vi "Kinesis - BNT - Set Circle Home Position.vi"() -> ()   [LabVIEW 2012]
doc: "Shows how to set and get the NanoTrak circle home position."
uses:
  U:/Kinesis LabVIEW Website Examples/Thorlabs.MotionControl.Controls.dll
  Thorlabs.MotionControl.Controls.dll
  U:/Kinesis LabVIEW Website Examples/Thorlabs.MotionControl.Benchtop.NanoTrakCLI.dll
  Thorlabs.MotionControl.Benchtop.NanoTrakCLI.dll
  U:/Kinesis LabVIEW Website Examples/Thorlabs.MotionControl.GenericNanoTrakCLI.dll
  Thorlabs.MotionControl.GenericNanoTrakCLI.dll
panel:
  in  "?":bool
  in  "Set Position":cluster{"HPosition":dbl, "VPosition":dbl}
  out "New Position":cluster{"HPosition":dbl, "VPosition":dbl}
  in  "?":bool
  out "Initial Position":cluster{"HPosition":dbl, "VPosition":dbl}
  in  "SerialNumber":string
  in  "BenchtopNanoTrakControl":refnum<k24>(container)
  # "Notes:"
  # "- Ensure that the appropriate .DLLs are copied into your Project Folder. Check that the correct bit type are used depending on your version of LabVIEW\ni.e. 32-bit or 64-bit.\n\n\n\n\n\n\n\n\n\n\n\n\n\n\n- Open the example VI through the LabVIEW Project Explorer to correctly load the User Interface from Thorlabs.MotionControl.Controls.dll."
  # "Thorlabs Hardware: BNT001/IR\nhttps://www.thorlabs.com/newgrouppage9.cfm?objectgroup_id=1194&pn=BNT001/IR"
  # "Description: This VI will enable you to set the Scanning Circle Home Position, throught the GetCircleHomePosition() method. \nHorizontal and Vertical positions can be adjusted in the range of 0 to 10 in NanoTrak Units."
  # "Instructions: \n1) Connect your BNT001 device to your PC & power the device. For full device setup, the device product manual can be found on our website here.\n - https://www.thorlabs.com/thorproduct.cfm?partnumber=BNT001/IR\n2) Enter the device serial number below.\n3) Click 'Run' in the LabVIEW Toolbar.\n5) Enter values for Horizontal & Vertical Position (0-10 NT Units). \n5) To end the Program, click 'END'."
  # "Example Image of .NET Controller - VI opened via Project Explorer/ not opened via Project Explorer"
  # "VI Not Opened via Project Explorer"
  # "VI Opened via Project Explorer"
  # "- To explore the range of methods available, please visit the .NET API, included with your Kinesis software.\n\n- For tips on building your own VIs with Thorlabs Motion Control Hardware, please see our LabVIEW Guide here.\nhttps://www.thorlabs.com/newgrouppage9.cfm?objectgroup_id=10285"
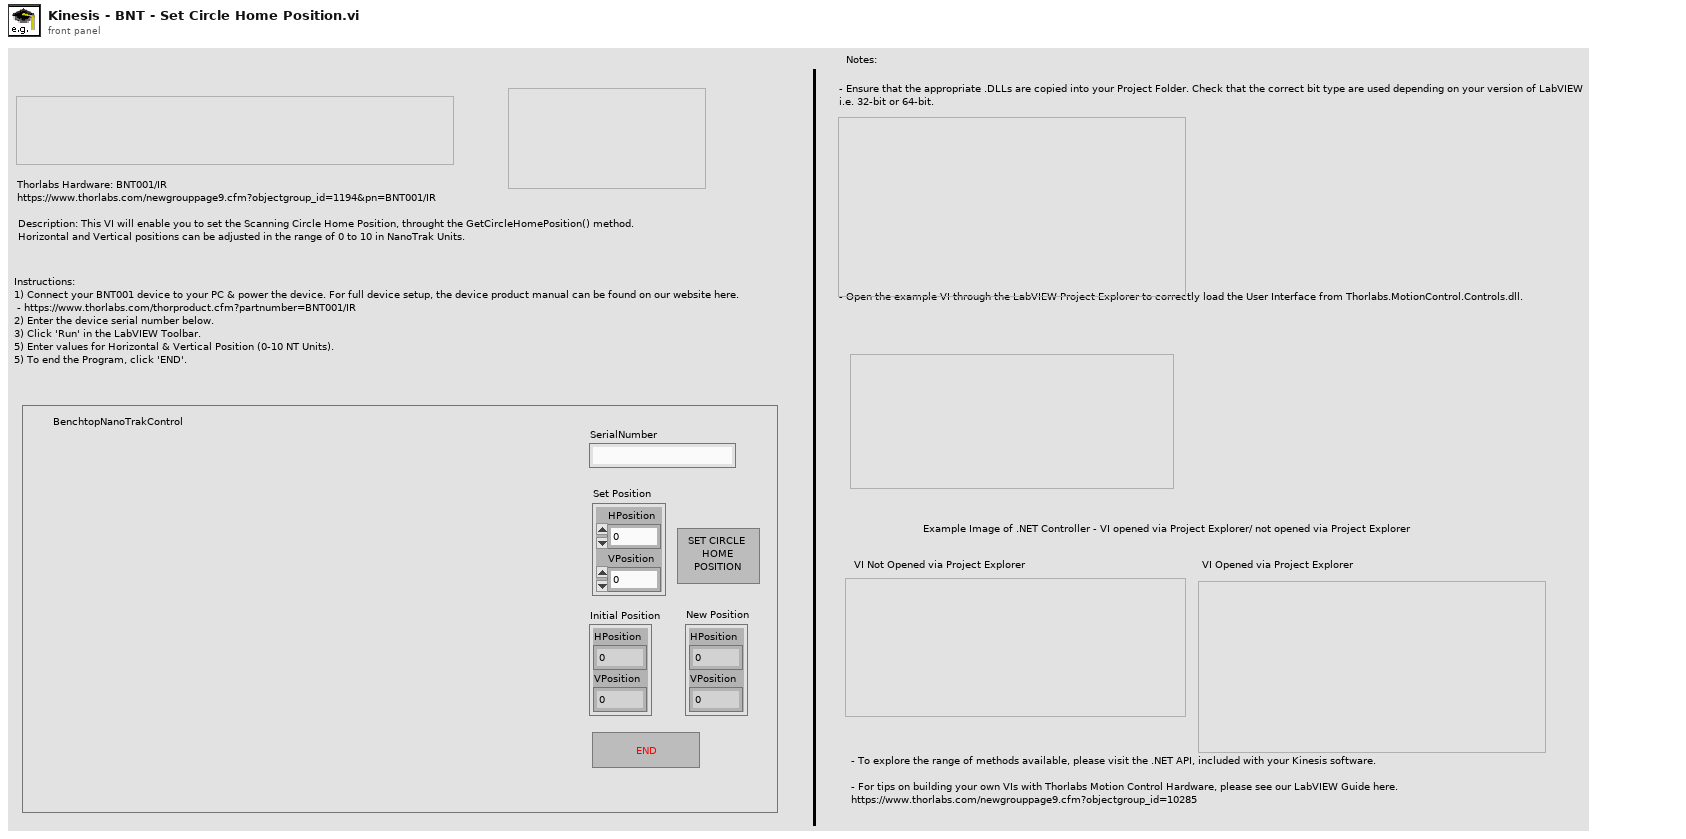
[diagram p1: front panel]
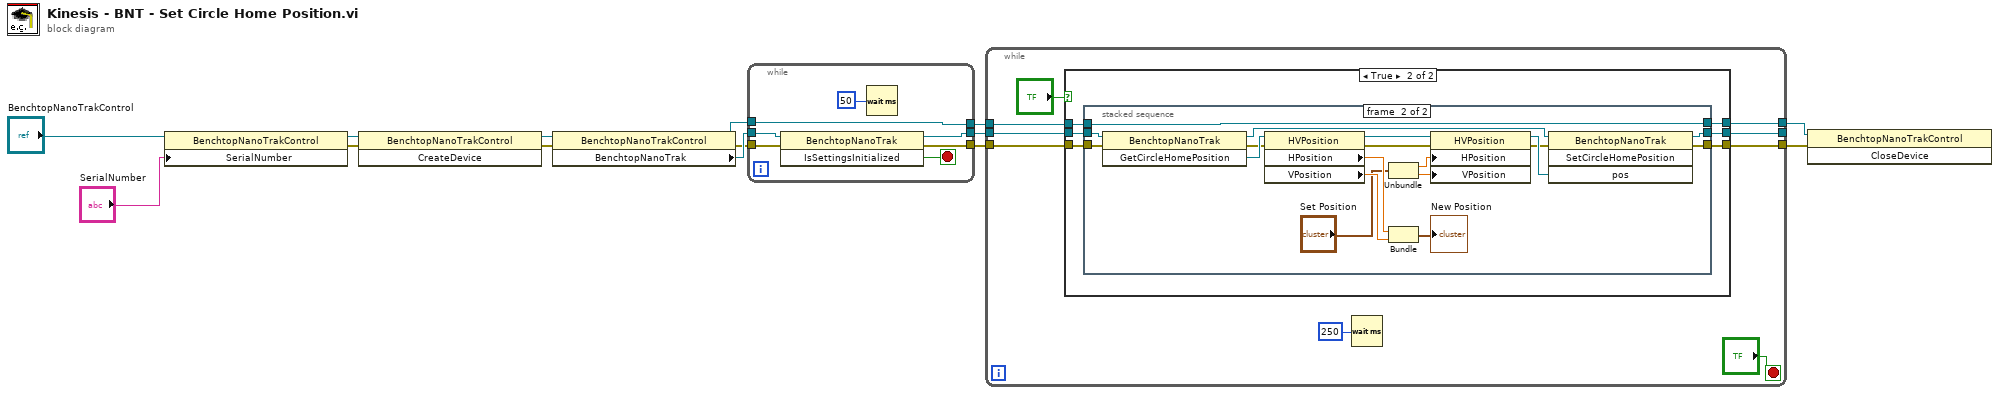
[diagram p0: block diagram]
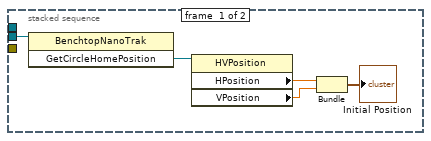
[diagram p3: hidden frame]
diagram:
  n1 = property class="BenchtopNanoTrakControl"(reference="BenchtopNanoTrakControl", "SerialNumber"="SerialNumber") -> (reference out=w12:refnum<k24>, error out=w7:errorcluster)  [unwired: 1 in]
  n2 = invoke class="BenchtopNanoTrakControl" method="CreateDevice"(reference=w12, error in=w7) -> (reference out=w11:refnum<k24>, error out=w8:errorcluster)  [unwired: 1 in, 1 out]
  n3 = property class="BenchtopNanoTrakControl"(reference=w11, error in=w8) -> (reference out=w1:refnum<k24>, error out=w9:errorcluster, "BenchtopNanoTrak"=w10:refnum<k24>)
  n4 = while {
    tunnel: w10 -> [w19]
    tunnel: [w18] -> w5
    tunnel: w9 -> [w17]
    tunnel: [w16] -> w6
    tunnel: [w15] -> w2
    tunnel: w1 -> [w15]
    stop <- w21 stop-if-true
    n5 = invoke class="BenchtopNanoTrak" method="IsSettingsInitialized"(reference=w19, error in=w17) -> (reference out=w18:refnum<k24>, error out=w16:errorcluster, "IsSettingsInitialized"=w21:bool)  [unwired: 1 in]
    n6 = Wait (ms)(milliseconds to wait=u32 50) -> ()  [unwired: 1 out]
  }
  n7 = while {
    tunnel: [w25] -> _
    tunnel: w6 -> [w28]
    tunnel: [w27] -> w4
    tunnel: w5 -> [w26]
    tunnel: [w24] -> w3
    tunnel: w2 -> [w23]
    stop <- "?" stop-if-true
    n8 = case shown="True" "?" {
      tunnel: w26 -> [w32 w39]
      tunnel: [w32 w38] -> w25
      tunnel: w28 -> [w33 w37]
      tunnel: [w33 w36] -> w27
      tunnel: [w31 w35] -> w24
      tunnel: w23 -> [w31 w34]
      frame False {
      }
      frame True {
        n9 = stacked-sequence {
          tunnel: w39 -> [w44 w58]
          tunnel: [_ w51] -> w38
          tunnel: w37 -> [_ w50]
          tunnel: [_ w46] -> w36
          tunnel: [_ w45] -> w35
          tunnel: w34 -> [_ w45]
          frame #0 {
            n10 = invoke class="BenchtopNanoTrak" method="GetCircleHomePosition"(reference=w44) -> ("GetCircleHomePosition"=w43:refnum<k24>)  [unwired: 2 in, 2 out]
            n11 = property class="HVPosition"(reference=w43) -> ("HPosition"=w42:dbl, "VPosition"=w41:dbl)  [unwired: 1 in, 2 out]
            n12 = Bundle("HPosition"=w42, "VPosition"=w41) -> (→"Initial Position":cluster{"HPosition":dbl, "VPosition":dbl})  [unwired: 1 in]
          }
          frame #1 {
            n13 = invoke class="BenchtopNanoTrak" method="GetCircleHomePosition"(reference=w58, error in=w50) -> (reference out=w52:refnum<k24>, error out=w49:errorcluster, "GetCircleHomePosition"=w62:refnum<k24>)  [unwired: 1 in]
            n14 = property class="HVPosition"(reference=w62, error in=w49) -> (reference out=w53:refnum<k24>, error out=w48:errorcluster, "HPosition"=w61:dbl, "VPosition"=w60:dbl)
            n15 = Unbundle("Set Position") -> ("HPosition"=w56:dbl, "VPosition"=w55:dbl)
            n16 = Bundle("HPosition"=w61, "VPosition"=w60) -> (→"New Position":cluster{"HPosition":dbl, "VPosition":dbl})  [unwired: 1 in]
            n17 = property class="HVPosition"(reference=w53, error in=w48, "HPosition"=w56, "VPosition"=w55) -> (reference out=w54:refnum<k24>, error out=w47:errorcluster)
            n18 = invoke class="BenchtopNanoTrak" method="SetCircleHomePosition"(reference=w52, error in=w47, "pos"=w54) -> (reference out=w51:refnum<k24>, error out=w46:errorcluster)  [unwired: 1 in, 2 out]
          }
        }
      }
    }
    n19 = Wait (ms)(milliseconds to wait=u32 250) -> ()  [unwired: 1 out]
  }
  n20 = invoke class="BenchtopNanoTrakControl" method="CloseDevice"(reference=w3, error in=w4) -> ()  [unwired: 1 in, 3 out]
